vi "Main.vi"() -> ()   [LabVIEW 2015]
uses:
  <vilib>/Utility/error.llb/Error Cluster From Error Code.vi
  <vilib>/ErrorRing/Error Ring.xnode
  Controller/TypeDefine/MainCtlsAndVIRef.ctl
  Controller/Panel_UI.lvclass
panel:
  in  "Indicate":bool
  in  "Panel":string
  in  "Reset":bool
  in  "查询数值":bool
  in  "Next Button":bool
  in  "Down Button":bool
  in  "Up Button":bool
  in  "Previous Button":bool
  in  "Log":bool
  in  "修改数值":bool
  in  "Stop":bool
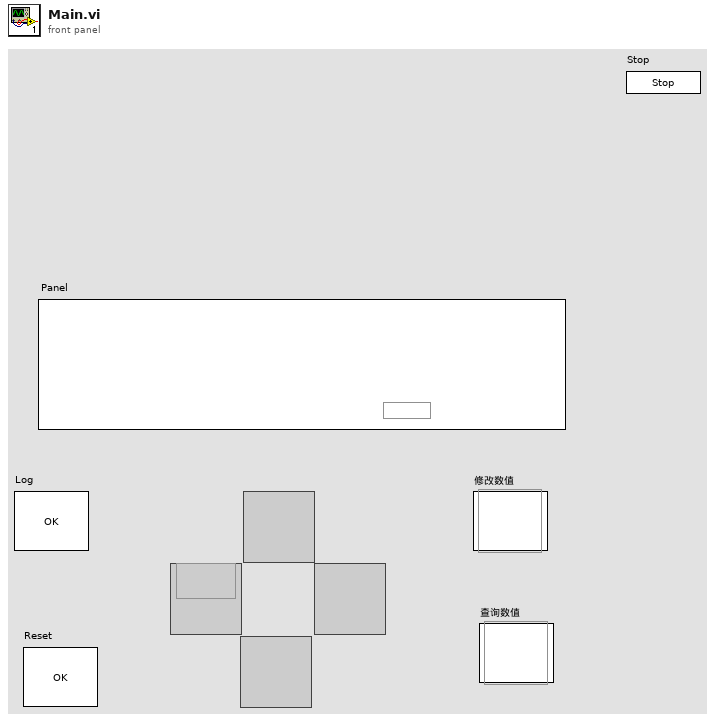
[diagram p1: front panel]
types:
  T1 = typedef "MainCtlsAndVIRef.ctl" = cluster{"Indicate":refnum<vi>, "Panel":refnum<vi>, "This VI":refnum<vi>}
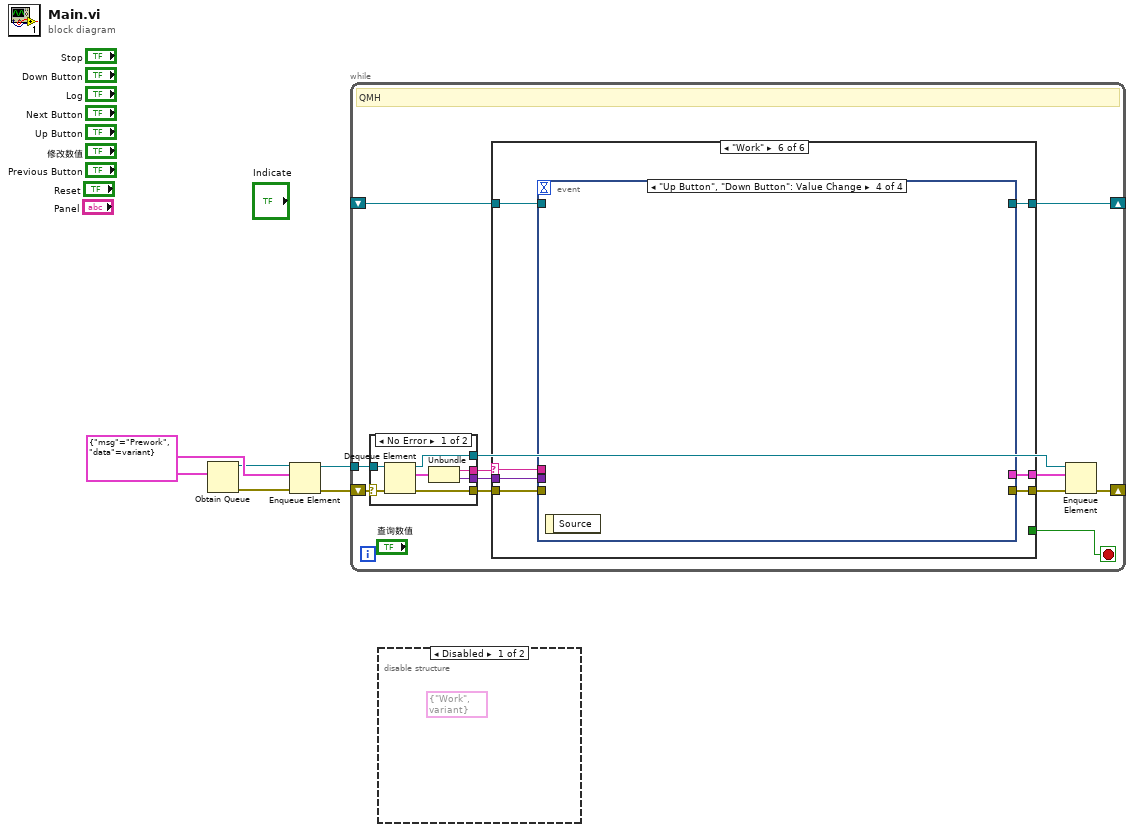
[diagram p0: block diagram]
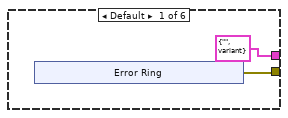
[diagram p3: hidden frame]
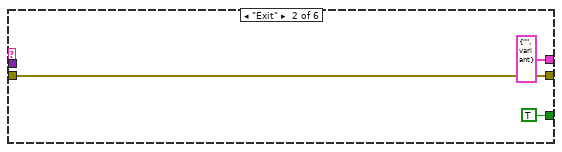
[diagram p4: hidden frame]
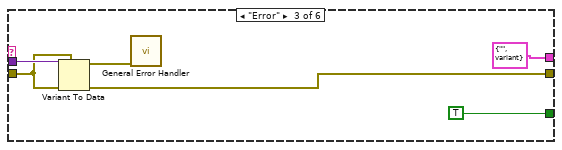
[diagram p5: hidden frame]
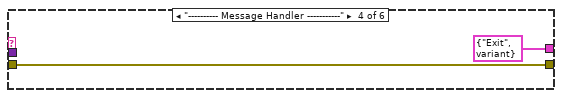
[diagram p6: hidden frame]
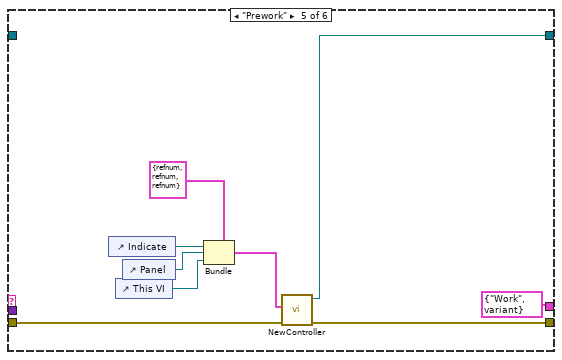
[diagram p7: hidden frame]
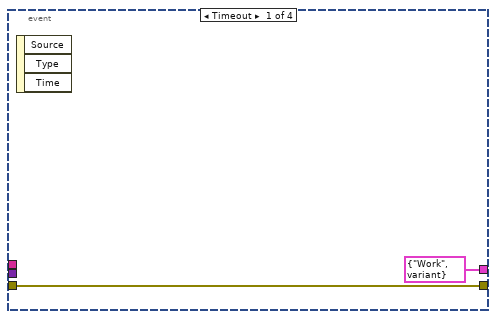
[diagram p8: hidden frame]
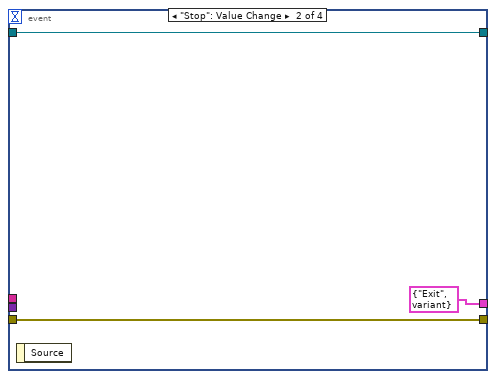
[diagram p9: hidden frame]
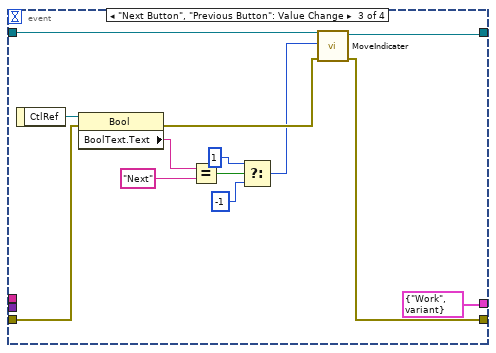
[diagram p10: hidden frame]
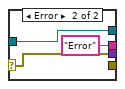
[diagram p11: hidden frame]
diagram:
  w3 = cluster{"msg":string, "data":variant} {"msg"="Prework", "data"=variant}
  n1 = Obtain Queue(element data type=w3) -> (queue out=w1:refnum<queue>, error out=w2:errorcluster)  [unwired: 4 in, 1 out]
  n2 = Enqueue Element(queue=w1, element=w3, error in (no error)=w2) -> (queue out=w4:refnum<queue>, error out=w5:errorcluster)  [unwired: 1 in, 1 out]
  n3 = while {
    tunnel: w4 -> [w16]
    shift-right: [w11] -> _
    shift-left: w5 -> [w17]
    shift-right: [w7] -> _
    shift-left: _ -> [w6]
    stop <- w8 stop-if-true
    # "QMH"
    n4 = case shown="No Error" w17 {
      selector: w17 -> [w75 w79]
      tunnel: w16 -> [w76 w77]
      tunnel: [w74 _] -> w15
      tunnel: [w72 "Error" ("msg")] -> w14
      tunnel: [w71 w79] -> w13
      tunnel: [w70 w77] -> w10
      frame No Error {
        n5 = Dequeue Element(queue=w76, error in (no error)=w75) -> (queue out=w70:refnum<queue>, element=w73:cluster{"msg":string, "data":variant}, error out=w74:errorcluster)  [unwired: 1 in, 1 out]
        n6 = Unbundle(w73) -> ("msg"=w72:string, "data"=w71:variant)
      }
      frame Error {
      }
    }
    n7 = case shown="\"Work\"" w14 {
      selector: w14 -> [_ _ _ _ _ w49]
      tunnel: w15 -> [_ w27 w32 w35 w39 w51]
      tunnel: w13 -> [_ _ w33 _ _ w50]
      tunnel: [w19 w27 w30 w35 w36 w48] -> w12
      tunnel: [cluster{"msg":string, "data":variant} {"msg"="", "data"=variant} cluster{"msg":string, "data":variant} {"msg"="", "data"=variant} cluster{"msg":string, "data":variant} {"msg"="", "data"=variant} cluster{"msg":string, "data":variant} {"msg"="Exit", "data"=variant} cluster{"msg":string, "data":variant} {"msg"="Work", "data"=variant} w47] -> w9
      tunnel: [_ TRUE TRUE _ _ _] -> w8
      tunnel: [_ _ _ _ w37 w45] -> w7
      tunnel: w6 -> [_ _ _ _ _ w46]
      frame Default {
        n8 = xnode "Error Ring"() -> ("error out"=w19:errorcluster)
      }
      frame "Exit" {
      }
      frame "Error" {
        n9 = Variant To Data(error in=w32, type=w32, Variant=w33) -> (data=w31:errorcluster, error out=w30:errorcluster)
        n10 = call <vilib>:"General Error Handler.vi"("error in (no error)"=w31) -> ()  [unwired: 10 in, 5 out]
      }
      frame "---------- Message Handler -----------" {
      }
      frame "Prework" {
        n11 = control-ref of="Indicate"() -> (w43:refnum<vi>)
        n12 = control-ref of="This VI"() -> (w41:refnum<vi>)
        n13 = control-ref of="Panel"() -> (w42:refnum<vi>)
        n14 = Bundle(cluster=T1 {"Indicate"=refnum, "Panel"=refnum, "This VI"=refnum}, "Indicate"=w43, "Panel"=w42, "This VI"=w41) -> (w38:T1)
        n15 = call "NewController.vi"("error in (no error)"=w39, "Controls"=w38) -> ("error out"=w36:errorcluster, "Panel_UI out"=w37:refnum<class "Panel_UI.lvclass">)  [unwired: 8 in]
      }
      frame "Work" {
        n16 = event shown="[3] \"Up Button\", \"Down Button\": Value Change" {
          selector: _ -> [_ _ _ _]
          dyn-events: _ -> [_ _ _ _]
          timeout: _ -> [_ _ _ _]
          tunnel: w51 -> [w53 w56 w68 _]
          tunnel: w50 -> [_ _ _ _]
          tunnel: w49 -> [_ _ _ _]
          tunnel: [w53 w56 w61 _] -> w48
          tunnel: [cluster{"msg":string, "data":variant} {"msg"="Work", "data"=variant} cluster{"msg":string, "data":variant} {"msg"="Exit", "data"=variant} cluster{"msg":string, "data":variant} {"msg"="Work", "data"=variant} _] -> w47
          tunnel: w46 -> [_ w54 w64 _]
          tunnel: [_ w54 w63 _] -> w45
          event Timeout {
            n17 = event-data() -> ()  [unwired: 1 in, 3 out]
          }
          event "Stop": Value Change {
            n18 = event-data() -> ()  [unwired: 1 in, 1 out]
          }
          event "Next Button", "Previous Button": Value Change {
            n19 = event-data() -> ("CtlRef"=w69:refnum<vi>)  [unwired: 1 in]
            n20 = property class="Bool"(reference=w69, error in=w68) -> (error out=w62:errorcluster, "BoolText.Text"=w67:string)  [unwired: 1 out]
            n21 = Equal?(x=w67, y="Next") -> (x = y?=w65:bool)
            n22 = Select(t=1, s=w65, f=-1) -> (s? t:f=w57:i32)
            n23 = call "MoveIndicater.vi"("error in (no error)"=w62, "Delta"=w57, "Panel_UI in"=w64) -> ("error out"=w61:errorcluster, "Panel_UI out"=w63:refnum<class "Panel_UI.lvclass">)  [unwired: 7 in]
          }
          event "Up Button", "Down Button": Value Change {
            n24 = event-data() -> ()  [unwired: 1 in, 1 out]
          }
        }
      }
    }
    n25 = Enqueue Element(queue=w10, element=w9, error in (no error)=w12) -> (error out=w11:errorcluster)  [unwired: 1 in, 2 out]
  }
  n26 = disable-structure shown="Disabled" {
    frame Disabled {
      (unwired) cluster{"msg":string, "data":variant} {"msg"="Work", "data"=variant}
    }
    frame Enabled {
    }
  }
